vi "array_maker.vi"(11 "row_number":i32) -> (3 "Array":i32[](array[numeric]))   [LabVIEW 2013]
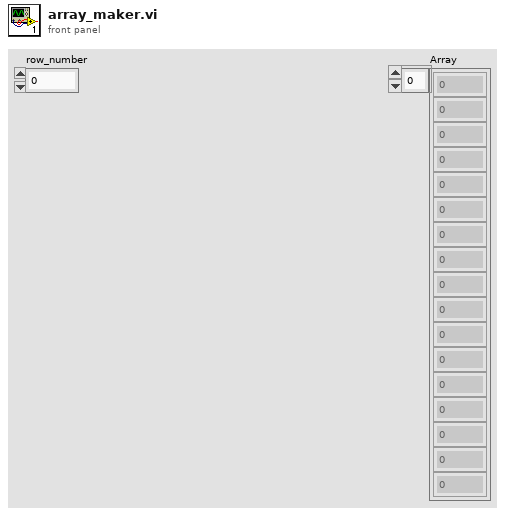
[diagram p1: front panel]
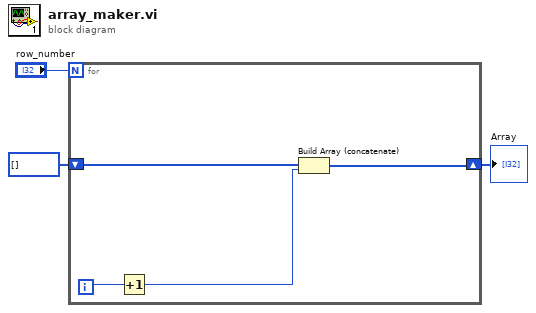
[diagram p0: block diagram]
diagram:
  n1 = for {
    N: "row_number" -> [_]
    shift-right: [w5] -> w1
    shift-left: i32[] [] -> [w4]
    i -> [w7]
    n2 = Increment(x=w7) -> (x+1=w6:i32)
    n3 = Build Array (concatenate)(w4, w6) -> (w5:i32[])
  }
  "Array" <- w1
